vi "滑移力复测判定.vi"(9 "压力判定项":string[][](table), 10 "拉力判定项":string[][](table), 11 "滑移力曲线":cluster{dbl[], dbl[]}[](graph)) -> (3 "判定":string[][](table))   [LabVIEW 2020]
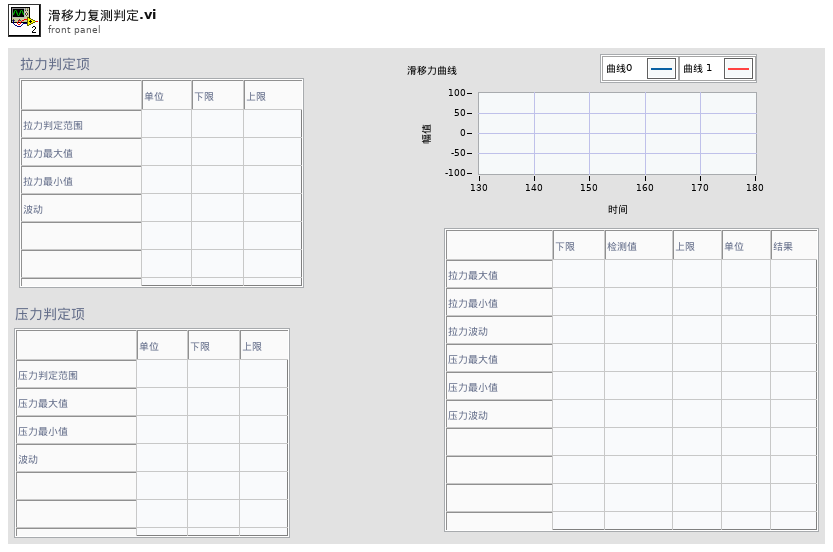
[diagram p1: front panel]
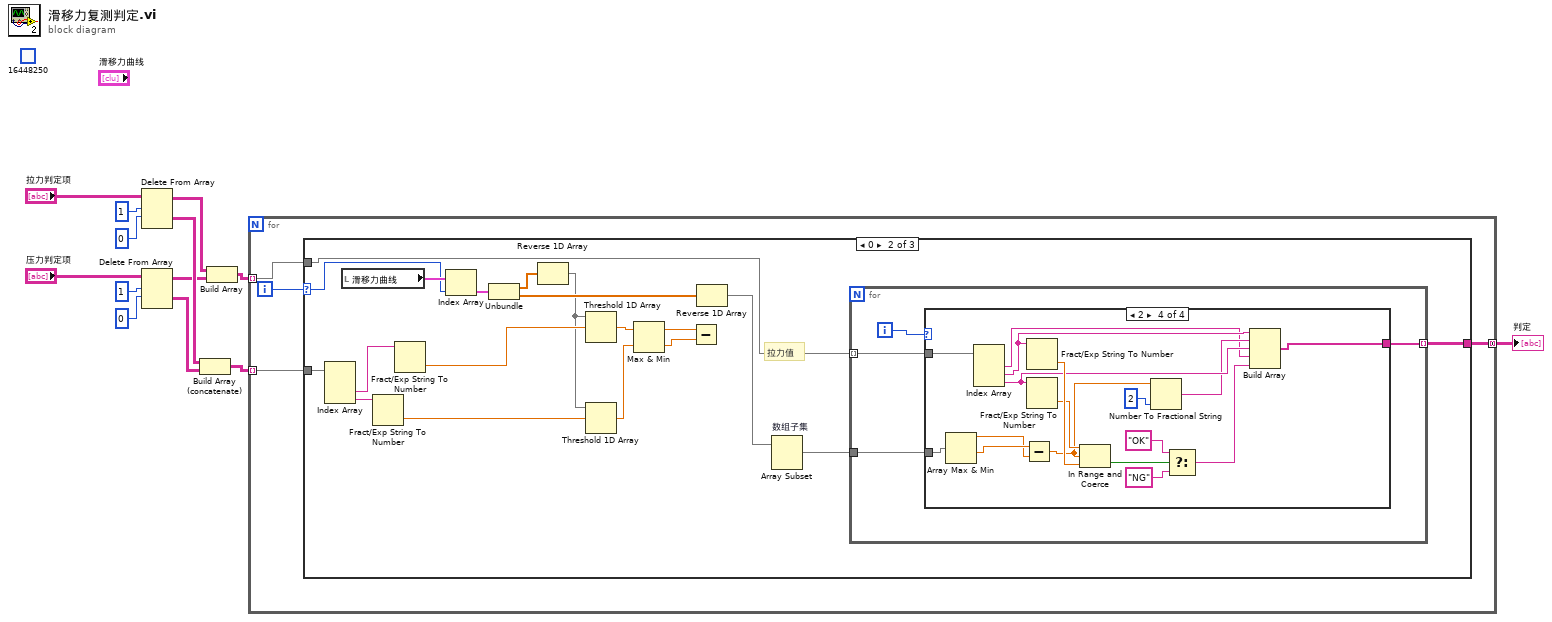
[diagram p0: block diagram]
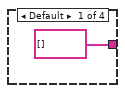
[diagram p3: hidden frame]
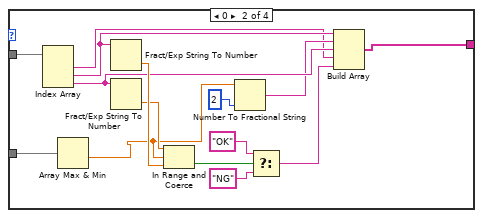
[diagram p4: hidden frame]
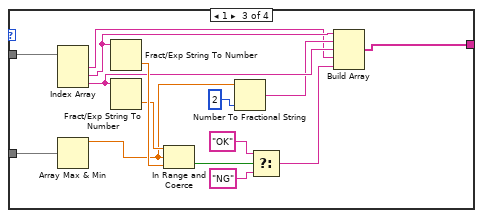
[diagram p5: hidden frame]
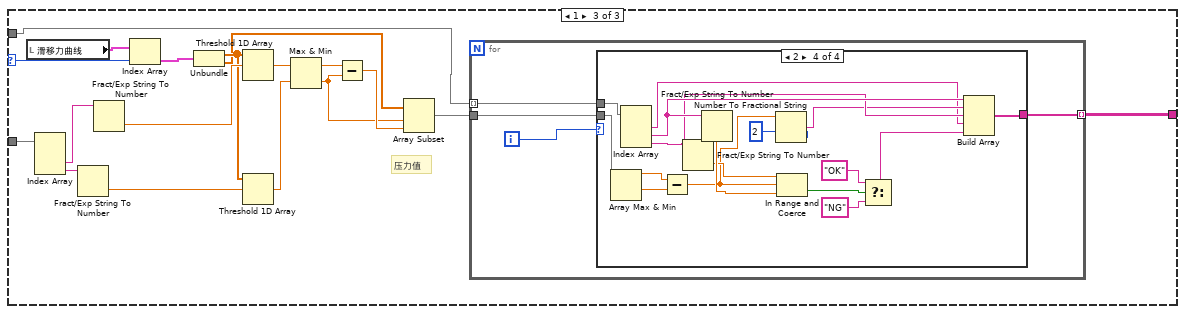
[diagram p6: hidden frame]
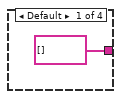
[diagram p7: hidden frame]
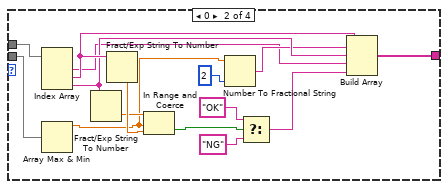
[diagram p8: hidden frame]
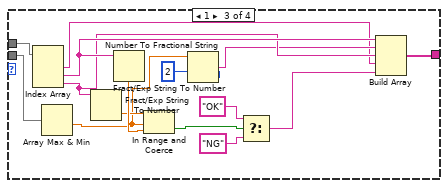
[diagram p9: hidden frame]
diagram:
  (unwired) u32 16448250
  n1 = Delete From Array ("删除数组元素")(array="拉力判定项", length=1 ("长度"), index (row)=0 ("索引 (行)")) -> (deleted portion=w7:string[][], array with subset deleted=w5:string[][])  [unwired: 1 in]
  n2 = Delete From Array(array="压力判定项", length=1 ("长度"), index (row)=0 ("索引 (行)")) -> (deleted portion=w6:string[][], array with subset deleted=w4:string[][])  [unwired: 1 in]
  n3 = Build Array (concatenate)(w7, w6) -> (w3:string[][])
  n4 = Build Array(w5, w4) -> (w2:string[][][])
  n5 = for {
    tunnel: w3 -> [w16] mode=indexing
    tunnel: w2 -> [w15] mode=indexing
    tunnel: [w14] -> w1 mode=concatenating
    i -> [w17]
    n6 = case shown="0" w17 {
      selector: w17 -> [_ w23 w91]
      tunnel: w16 -> [_ w32 w104]
      tunnel: w15 -> [_ w26 w96]
      tunnel: [_ w24 w92] -> w14
      frame Default {
      }
      frame 0 {
        # "拉力值"
        n7 = Index Array(array=w32) -> (element #2=w31:string, element #3=w30:string)  [unwired: 3 in, 1 out]
        n8 = local read "滑移力曲线"() -> (w36:cluster{dbl[], dbl[]}[])
        n9 = Fract/Exp String To Number ("分数/指数字符串至数值转换")(string=w30) -> (number=w28:dbl)  [unwired: 3 in, 1 out]
        n10 = Fract/Exp String To Number(string=w31) -> (number=w29:dbl)  [unwired: 3 in, 1 out]
        n11 = Index Array(array=w36, index=w23) -> (element=w35:cluster{dbl[], dbl[]})
        n12 = Unbundle(w35) -> (w34:dbl[], w33:dbl[])
        n13 = Reverse 1D Array(array=w34) -> (reversed array=w27:dbl[])
        n14 = Threshold 1D Array ("以阈值插值一维数组")(2:w29, 3:w27) -> (0:w20:dbl)  [unwired: 1 in]
        n15 = Threshold 1D Array(2:w28, 3:w27) -> (0:w19:dbl)  [unwired: 1 in]
        n16 = Max & Min ("最大值与最小值")(x=w20, y=w19) -> (max(x,y)=w22:dbl, min(x,y)=w21:dbl)
        n17 = Subtract(x=w22, y=w21) -> ()  [unwired: 1 out]
        n18 = Reverse 1D Array(array=w33) -> (reversed array=w18:dbl[])
        n19 = Array Subset "数组子集"(array=w18) -> (w25:dbl[])  [unwired: 2 in]
        n20 = for {
          tunnel: w26 -> [w39] mode=indexing
          tunnel: w25 -> [w38]
          tunnel: [w37] -> w24 mode=indexing
          i -> [w40]
          n21 = case shown="2" w40 {
            tunnel: w39 -> [_ w56 w71 w88]
            tunnel: w38 -> [_ w53 w68 w85]
            tunnel: [string[] [] w43 w58 w75] -> w37
            frame Default {
            }
            frame 0 {
              n22 = Index Array(array=w56) -> (element #1=w48:string, element #2=w52:string, element #3=w51:string)  [unwired: 3 in]
              n23 = Array Max & Min(array=w53) -> (min value=w42:dbl)  [unwired: 3 out]
              n24 = Fract/Exp String To Number(string=w52) -> (number=w55:dbl)  [unwired: 3 in, 1 out]
              n25 = Fract/Exp String To Number(string=w51) -> (number=w54:dbl)  [unwired: 3 in, 1 out]
              n26 = In Range and Coerce(upper limit=w54, x=w42, lower limit=w55) -> (In Range?=w47:bool)  [unwired: 1 out]
              n27 = Number To Fractional String(number=w42, precision (6)=i16 2 ("精度(6)")) -> (F-format string=w49:string)  [unwired: 2 in]
              n28 = Select(t="OK", s=w47, f="NG") -> (s? t:f=w44:string)
              n29 = Build Array(w52, w49, w51, w48, w44) -> (w43:string[])
            }
            frame 1 {
              n30 = Index Array(array=w71) -> (element #1=w63:string, element #2=w67:string, element #3=w66:string)  [unwired: 3 in]
              n31 = Array Max & Min(array=w68) -> (max value=w57:dbl)  [unwired: 3 out]
              n32 = Fract/Exp String To Number(string=w67) -> (number=w70:dbl)  [unwired: 3 in, 1 out]
              n33 = Fract/Exp String To Number(string=w66) -> (number=w69:dbl)  [unwired: 3 in, 1 out]
              n34 = In Range and Coerce(upper limit=w69, x=w57, lower limit=w70) -> (In Range?=w62:bool)  [unwired: 1 out]
              n35 = Number To Fractional String(number=w57, precision (6)=i16 2 ("精度(6)")) -> (F-format string=w64:string)  [unwired: 2 in]
              n36 = Select(t="OK", s=w62, f="NG") -> (s? t:f=w59:string)
              n37 = Build Array(w67, w64, w66, w63, w59) -> (w58:string[])
            }
            frame 2 {
              n38 = Array Max & Min(array=w85) -> (max value=w73:dbl, min value=w74:dbl)  [unwired: 2 out]
              n39 = Index Array(array=w88) -> (element #1=w80:string, element #2=w84:string, element #3=w83:string)  [unwired: 3 in]
              n40 = Subtract(x=w74, y=w73) -> (x-y=w72:dbl)
              n41 = Fract/Exp String To Number(string=w84) -> (number=w87:dbl)  [unwired: 3 in, 1 out]
              n42 = Fract/Exp String To Number(string=w83) -> (number=w86:dbl)  [unwired: 3 in, 1 out]
              n43 = In Range and Coerce(upper limit=w86, x=w72, lower limit=w87) -> (In Range?=w79:bool)  [unwired: 1 out]
              n44 = Number To Fractional String(number=w72, precision (6)=i16 2 ("精度(6)")) -> (F-format string=w81:string)  [unwired: 2 in]
              n45 = Select(t="OK", s=w79, f="NG") -> (s? t:f=w76:string)
              n46 = Build Array(w84, w81, w83, w80, w76) -> (w75:string[])
            }
          }
        }
      }
      frame 1 {
        # "压力值"
        n47 = local read "滑移力曲线"() -> (w106:cluster{dbl[], dbl[]}[])
        n48 = Index Array(array=w104) -> (element #2=w103:string, element #3=w102:string)  [unwired: 3 in, 1 out]
        n49 = Fract/Exp String To Number(string=w102) -> (number=w100:dbl)  [unwired: 3 in, 1 out]
        n50 = Fract/Exp String To Number(string=w103) -> (number=w101:dbl)  [unwired: 3 in, 1 out]
        n51 = Index Array(array=w106, index=w91) -> (element=w105:cluster{dbl[], dbl[]})
        n52 = Unbundle(w105) -> (w99:dbl[], w95:dbl[])
        n53 = Threshold 1D Array(2:w101, 3:w99) -> (0:w98:dbl)  [unwired: 1 in]
        n54 = Threshold 1D Array(2:w100, 3:w99) -> (0:w97:dbl)  [unwired: 1 in]
        n55 = Max & Min(x=w98, y=w97) -> (max(x,y)=w90:dbl, min(x,y)=w89:dbl)
        n56 = Subtract(x=w90, y=w89) -> (x-y=w94:dbl)
        n57 = Array Subset(array=w95, index=w89, length=w94) -> (w93:dbl[])
        n58 = for {
          tunnel: w96 -> [w109] mode=indexing
          tunnel: w93 -> [w108]
          tunnel: [w107] -> w92 mode=indexing
          i -> [w110]
          n59 = case shown="2" w110 {
            tunnel: w109 -> [_ w126 w141 w158]
            tunnel: w108 -> [_ w123 w138 w155]
            tunnel: [string[] [] w112 w128 w145] -> w107
            frame Default {
            }
            frame 0 {
              n60 = Index Array(array=w126) -> (element #1=w117:string, element #2=w122:string, element #3=w121:string)  [unwired: 3 in]
              n61 = Array Max & Min(array=w123) -> (max value=w120:dbl)  [unwired: 3 out]
              n62 = Fract/Exp String To Number(string=w121) -> (number=w124:dbl)  [unwired: 3 in, 1 out]
              n63 = Fract/Exp String To Number(string=w122) -> (number=w125:dbl)  [unwired: 3 in, 1 out]
              n64 = In Range and Coerce(upper limit=w124, x=w120, lower limit=w125) -> (In Range?=w116:bool)  [unwired: 1 out]
              n65 = Number To Fractional String ("数值至小数字符串转换")(number=w120, precision (6)=i16 2 ("精度(6)")) -> (F-format string=w118:string)  [unwired: 2 in]
              n66 = Select(t="OK", s=w116, f="NG") -> (s? t:f=w113:string)
              n67 = Build Array(w122, w118, w121, w117, w113) -> (w112:string[])
            }
            frame 1 {
              n68 = Index Array(array=w141) -> (element #1=w133:string, element #2=w137:string, element #3=w136:string)  [unwired: 3 in]
              n69 = Array Max & Min(array=w138) -> (min value=w127:dbl)  [unwired: 3 out]
              n70 = Fract/Exp String To Number(string=w136) -> (number=w139:dbl)  [unwired: 3 in, 1 out]
              n71 = Fract/Exp String To Number(string=w137) -> (number=w140:dbl)  [unwired: 3 in, 1 out]
              n72 = In Range and Coerce(upper limit=w139, x=w127, lower limit=w140) -> (In Range?=w132:bool)  [unwired: 1 out]
              n73 = Number To Fractional String(number=w127, precision (6)=i16 2 ("精度(6)")) -> (F-format string=w134:string)  [unwired: 2 in]
              n74 = Select(t="OK", s=w132, f="NG") -> (s? t:f=w129:string)
              n75 = Build Array(w137, w134, w136, w133, w129) -> (w128:string[])
            }
            frame 2 {
              n76 = Array Max & Min(array=w155) -> (max value=w143:dbl, min value=w144:dbl)  [unwired: 2 out]
              n77 = Index Array(array=w158) -> (element #1=w150:string, element #2=w154:string, element #3=w153:string)  [unwired: 3 in]
              n78 = Subtract(x=w143, y=w144) -> (x-y=w142:dbl)
              n79 = Fract/Exp String To Number(string=w153) -> (number=w156:dbl)  [unwired: 3 in, 1 out]
              n80 = Fract/Exp String To Number(string=w154) -> (number=w157:dbl)  [unwired: 3 in, 1 out]
              n81 = Number To Fractional String(number=w142, precision (6)=i16 2 ("精度(6)")) -> (F-format string=w151:string)  [unwired: 2 in]
              n82 = In Range and Coerce(upper limit=w156, x=w142, lower limit=w157) -> (In Range?=w149:bool)  [unwired: 1 out]
              n83 = Select(t="OK", s=w149, f="NG") -> (s? t:f=w146:string)
              n84 = Build Array(w154, w151, w153, w150, w146) -> (w145:string[])
            }
          }
        }
      }
    }
  }
  "判定" <- w1
